vi "getFPGA.vi"(11 "HealthAndStatusControlFIFO in":refnum<class "HealthAndStatusControlFIFO.lvclass">) -> (2 "FPGA":refnum<class "FPGA.lvclass">, 3 "HealthAndStatusControlFIFO out":refnum<class "HealthAndStatusControlFIFO.lvclass">)   [LabVIEW 2016, in "HealthAndStatusControlFIFO.lvclass"]
uses:
  HealthAndStatusControlFIFO.lvclass
  FPGA/FPGA.lvclass
  HealthAndStatusControlFIFO.lvclass/HealthAndStatusControlFIFO.ctl
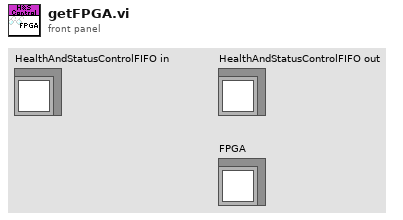
[diagram p1: front panel]
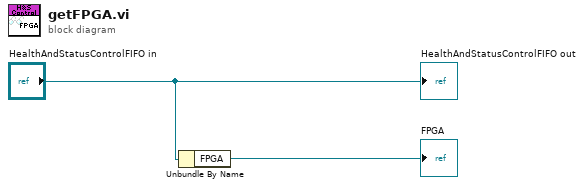
[diagram p0: block diagram]
diagram:
  n1 = Unbundle By Name("HealthAndStatusControlFIFO in") -> ("FPGA"=→"FPGA":refnum<class "FPGA.lvclass">)
  "HealthAndStatusControlFIFO out" <- "HealthAndStatusControlFIFO in"
